vi "AD5781VoltTransferFunc.vi"(8 "act Step 18 Bit":u32=16 max=262143 format="%018b", 10 "VREFN":dbl, 11 "VREFP":dbl) -> (3 "VOUT":dbl)   [LabVIEW 2014]
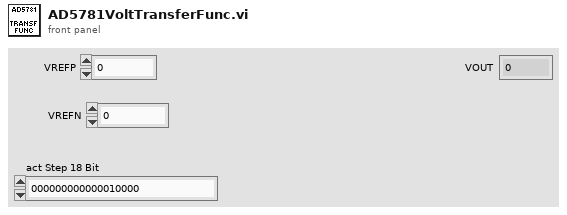
[diagram p1: front panel]
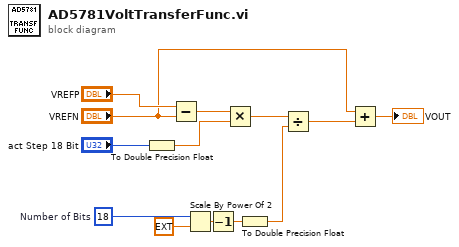
[diagram p0: block diagram]
diagram:
  w8 = u32 18  # Number of Bits
  n1 = To Double Precision Float(number="act Step 18 Bit") -> (double precision float=w9:dbl)
  n2 = Subtract(x="VREFP", y="VREFN") -> (x-y=w12:dbl)
  n3 = Scale By Power Of 2(n=w8, x=ext 1.0) -> (x*2^n=w6:ext)
  n4 = Decrement(x=w6) -> (x-1=w5:ext)
  n5 = Multiply(x=w12, y=w9) -> (x*y=w11:dbl)
  n6 = To Double Precision Float(number=w5) -> (double precision float=w4:dbl)
  n7 = Divide(x=w11, y=w4) -> (x/y=w3:dbl)
  n8 = Add(x="VREFN", y=w3) -> (x+y=→"VOUT":dbl)
